vi "Power Qualtiy - 8.vi"() -> ()   [LabVIEW 2015]
uses:
  <vilib>/addons/Electrical Power/Basic/Measurement/RMS (N Channels).vi
  <vilib>/addons/Electrical Power/Basic/Measurement/Power (1 Channel).vi
  <vilib>/Utility/file.llb/Write Delimited Spreadsheet (DBL).vi
  <vilib>/addons/Electrical Power/Basic/NI_EP_Basic.lvlib
panel:
  out "Active Power":dbl[](array[numeric])
  out "Current":dbl
  out "Power Factor":dbl[](array[numeric])
  out "IHD 7":dbl
  out "IHD 5":dbl
  out "IHD 3":dbl
  out "IHD 1":dbl
  out "Voltage Waveform":dynamicdata(graph)
  out "Current Waveform":dynamicdata(graph)
  out "Current":dbl(knob) scale=0.0..10.0
  out "Voltage":dbl(knob) scale=0.0..250.0
  out "THD":dbl
  out "Current Harmonics":dynamicdata(graph)
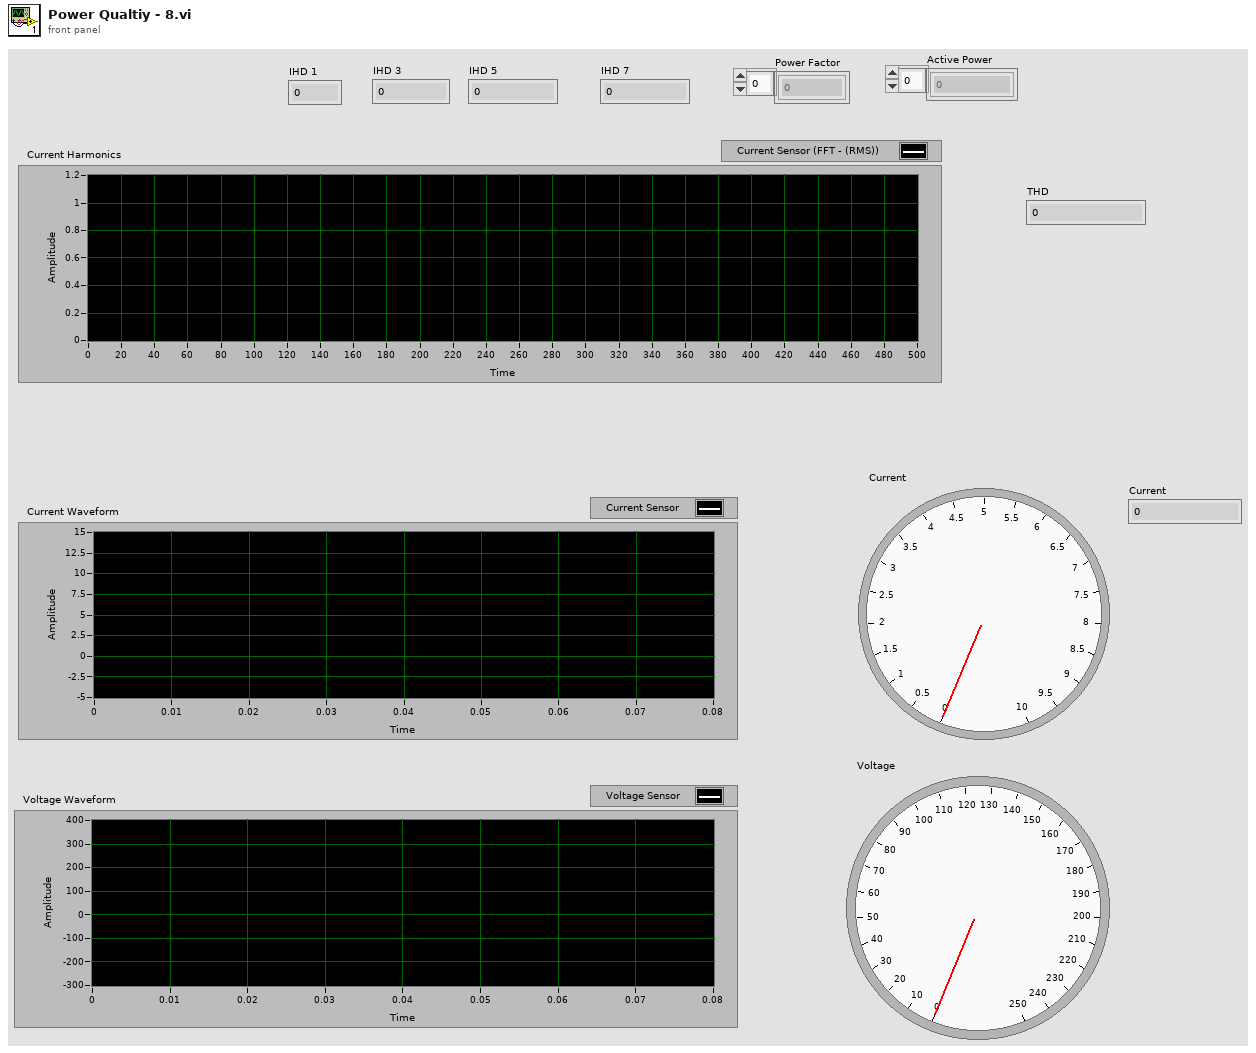
[diagram p1: front panel]
types:
  T1 = typedef "NI_EP_Basic.lvlib/basic_Power Value.ctl" = cluster{"active power [W]":dbl, "apparent power [VA]":dbl, "reactive power [VAR]":dbl, "power factor":dbl}
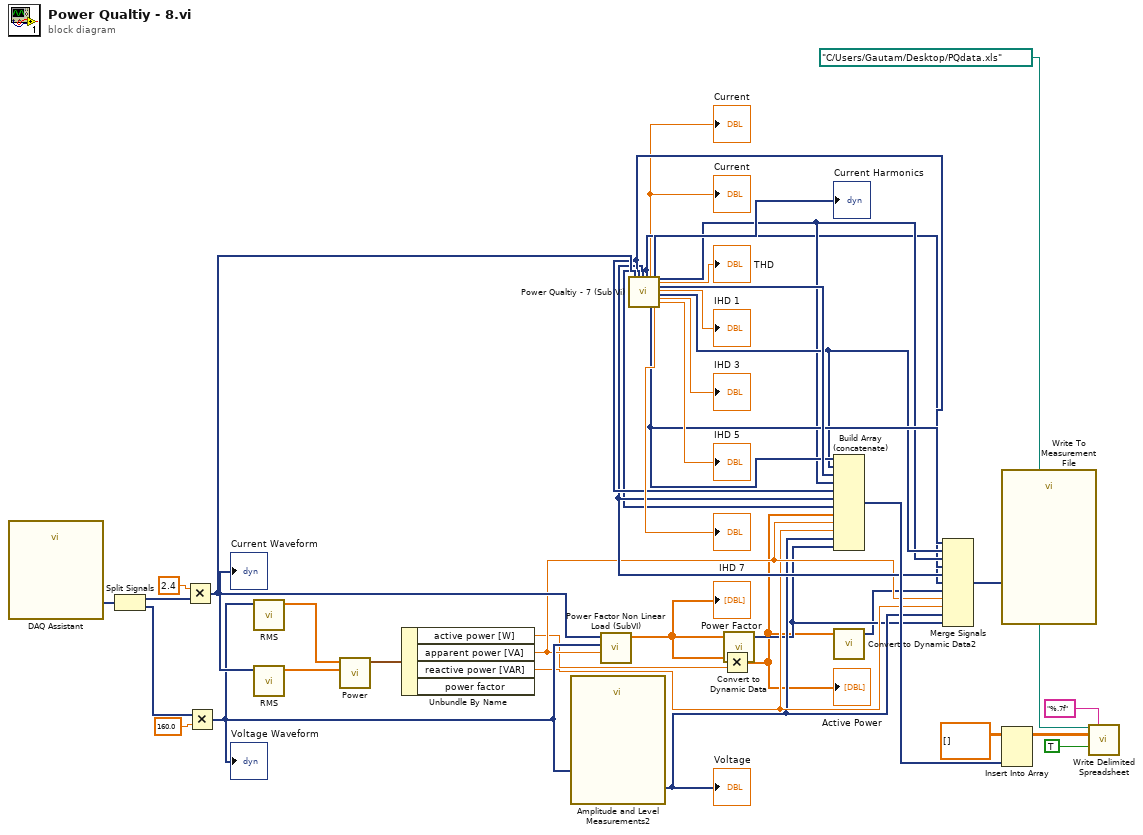
[diagram p0: block diagram]
diagram:
  n1 = call "DAQ Assistant"() -> ("data"=w39:dynamicdata)  [unwired: 17 in, 2 out]
  n2 = Split Signals(w39) -> (w38:dynamicdata, w37:dynamicdata)  [unwired: 2 in]
  n3 = Multiply(x=2.4, y=w38) -> (x*y=w25:dynamicdata)
  "Current Waveform" <- w25
  n4 = Multiply(x=w37, y=160.0) -> (x*y=w24:dynamicdata)
  "Voltage Waveform" <- w24
  n5 = call-poly <vilib>:"RMS.vi"("waveforms"=w24) -> ("RMS values"=w34:dbl[])  [unwired: 9 in, 1 out]
  n6 = call-poly <vilib>:"RMS.vi"("waveforms"=w25) -> ("RMS values"=w33:dbl[])  [unwired: 9 in, 1 out]
  n7 = call-poly <vilib>:"Power.vi"("current waveform"=w33, "voltage waveform"=w34) -> ("power value"=w32:T1)  [unwired: 8 in, 1 out]
  n8 = Unbundle By Name(w32) -> ("active power [W]"=w3:dbl, "apparent power [VA]"=w11:dbl, "reactive power [VAR]"=w10:dbl)  [unwired: 1 out]
  n9 = call "Amplitude and Level Measurements2"("Signals"=w24) -> ("RMS"=w9:dynamicdata)  [unwired: 13 in, 1 out]
  "Voltage" <- w9
  n10 = call "Power Factor Non Linear Load (SubVI).vi"("apparent power [VA]"=w11, "Dynamic Data"=w24, "Dynamic Data 2"=w25) -> ("Power Factor"=w2:dbl[])  [unwired: 8 in]
  "Power Factor" <- w2
  n11 = call "Power Qualtiy - 7 (Sub Vi).vi"("Dynamic Data 6"=w25) -> ("Dynamic Data 2"=w14:dynamicdata, "Dynamic Data"=w13:dynamicdata, "Dynamic Data 4"=w12:dynamicdata, "Current"=→"Current" →"Current":dbl, "RMS"=w17:dynamicdata, "Current Harmonics"=→"Current Harmonics":dynamicdata, "IHD 7"=→"IHD 7":dbl, "Dynamic Data 3"=w15:dynamicdata, "THD"=→"THD":dbl, "Dynamic Data 5"=w23:dynamicdata, "IHD 1"=→"IHD 1":dbl, "THD 2"=w16:dynamicdata, "IHD 3"=→"IHD 3":dbl, "IHD 5"=→"IHD 5":dbl)  [unwired: 12 in, 1 out]
  n12 = Multiply(x=w2, y=w3) -> (x*y=w4:dbl[])
  "Active Power" <- w4
  n13 = call "Convert to Dynamic Data"("Array"=w2) -> ("Dynamic Data Type"=w8:dynamicdata)  [unwired: 3 in]
  n14 = Build Array (concatenate)(w17, w16, w23, w15, w14, w13, w12, w4, w11, w10, w9, w8) -> (w22:dynamicdata[])
  n15 = call "Convert to Dynamic Data2"("Array"=w4) -> ("Dynamic Data Type"=w1:dynamicdata)  [unwired: 3 in]
  n16 = Merge Signals(w17, w16, w15, w14, w13, w12, w1, w11, w10, w9, w8) -> (w7:dynamicdata)
  n17 = call "Write To Measurement File"("Signals"=w7) -> ()  [unwired: 16 in, 3 out]
  n18 = Insert Into Array(array=dbl[][] [], new element=w22) -> (w18:dbl[][])  [unwired: 2 in]
  n19 = call-poly <vilib>:"Write Delimited Spreadsheet.vi"("file path (dialog if empty)"=path "C:/Users/Gautam/Desktop/PQdata.xls", "format (%.3f)"="%.7f", "2D data"=w18, "append to file? (F)"=TRUE) -> ()  [unwired: 10 in, 2 out]
